vi "Read ActiveFlag.vi"(8 "error in (no error)":errorcluster, 11 "ESP301 in":refnum<class "ESP301.lvclass">) -> (0 "error out":errorcluster, 2 "ActiveFlag":cluster{"Axis 1":T1, "Axis 2":T1, "Axis 3":T1}, 3 "ESP301 out":refnum<class "ESP301.lvclass">)   [LabVIEW 2020, in "ESP301.lvclass"]
uses:
  ESP301.lvclass
  activeflag.ctl
  ESP301.lvclass/ESP301.ctl
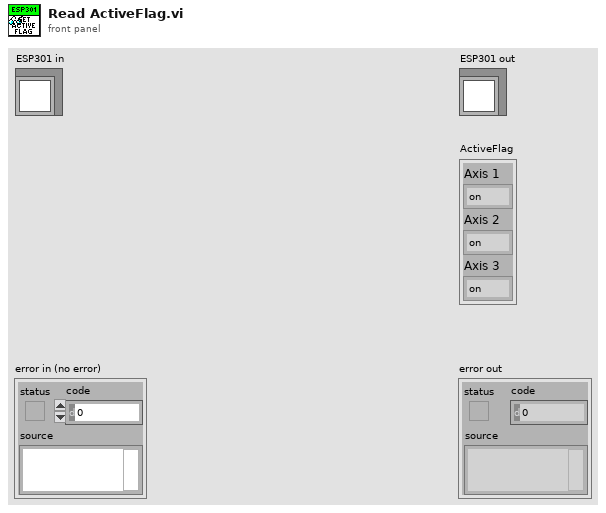
[diagram p1: front panel]
types:
  T1 = typedef "activeflag.ctl" = enum16{"on", "off", "n/a"}
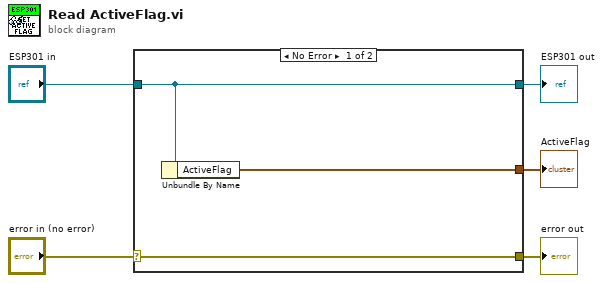
[diagram p0: block diagram]
diagram:
  n1 = case shown="No Error" "error in (no error)" {
    selector: "error in (no error)" -> [w8 w9]
    tunnel: [w8 w9] -> w4
    tunnel: [w7 w10] -> w2
    tunnel: "ESP301 in" -> [w7 w10]
    tunnel: [w6 _] -> w1
    frame No Error {
      n2 = Unbundle By Name(w7) -> ("ActiveFlag"=w6:cluster{"Axis 1":T1, "Axis 2":T1, "Axis 3":T1})
    }
    frame Error {
    }
  }
  "error out" <- w4
  "ESP301 out" <- w2
  "ActiveFlag" <- w1
